vi "test_Add Command_Channel Reference Error.vi"(8 "error in (no error)":errorcluster, 11 "TestCase in":refnum<class "Instrument Addon Scripting API Messages Unit Tests.lvclass">) -> (0 "error out":errorcluster, 3 "TestCase out":refnum<class "Instrument Addon Scripting API Messages Unit Tests.lvclass">)   [LabVIEW 2019, in "Instrument Addon Scripting API Messages Unit Tests.lvclass"]
uses:
  Instrument Addon Scripting API Messages Unit Tests.lvclass
  APIs/Scripting API/TypeDefs/Command Settings.ctl
  <vilib>/NI VeriStand/Custom Device API/Custom Device Item Ref.ctl
  APIs/Scripting API/TypeDefs/Padding.ctl
  Instrument Addon Scripting API Messages Unit Tests.lvclass/Instrument Addon Scripting API Messages Unit Tests.ctl
  Addon/Addon Shared/SubVIs/Constants.vi
  <vilib>/NI/NI VeriStand Advanced SysDef API/_SubVIs/SysDef.Search.GUID.vi
  <vilib>/addons/_JKI Toolkits/VI Tester/TestCase.llb/TestCase.lvclass
  Instrument Addon Scripting API Test Assets/Instrument Addon Scripting API Test Assets.lvclass
  <vilib>/NI/NI VeriStand Advanced SysDef API/SysDef API/Advanced System Definition.lvlib
  Addon/Addon Shared/Instrument Addon Shared.lvlib
  <vilib>/NI VeriStand/Custom Device API/Custom Device API.lvlib
  APIs/Scripting API/Instrument Addon Scripting API.lvlib
  C:/Program Files (x86)/National Instruments/LabVIEW 2019/vi.lib/addons/_JKI Toolkits/VI Tester/TestCase.llb/TestCase.lvclass
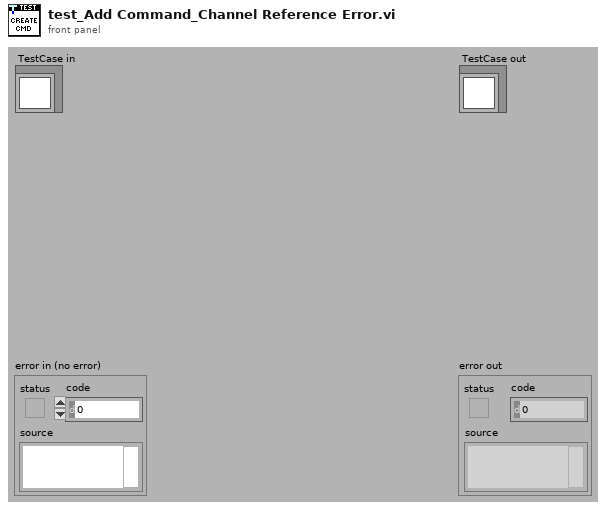
[diagram p1: front panel]
types:
  T1 = typedef "Custom Device API.lvlib/Custom Device Item Ref.ctl" = u64
  T2 = cluster{"Variable Name":string, "Channel Ref in":T1}
  T3 = typedef "Instrument Addon Scripting API.lvlib/Command Settings.ctl" = cluster{"Command Format":string, "Linked Channels":cluster{"Variable Name":string, "Channel Ref in":T1}[], "Use Padding?":bool, "Padding":T4}
  T4 = typedef "Instrument Addon Scripting API.lvlib/Padding.ctl" = cluster{"Pad Value":u8, "Length":u32}
  T5 = cluster{"Variable Name":string, "Channel Ref in":T1}[]
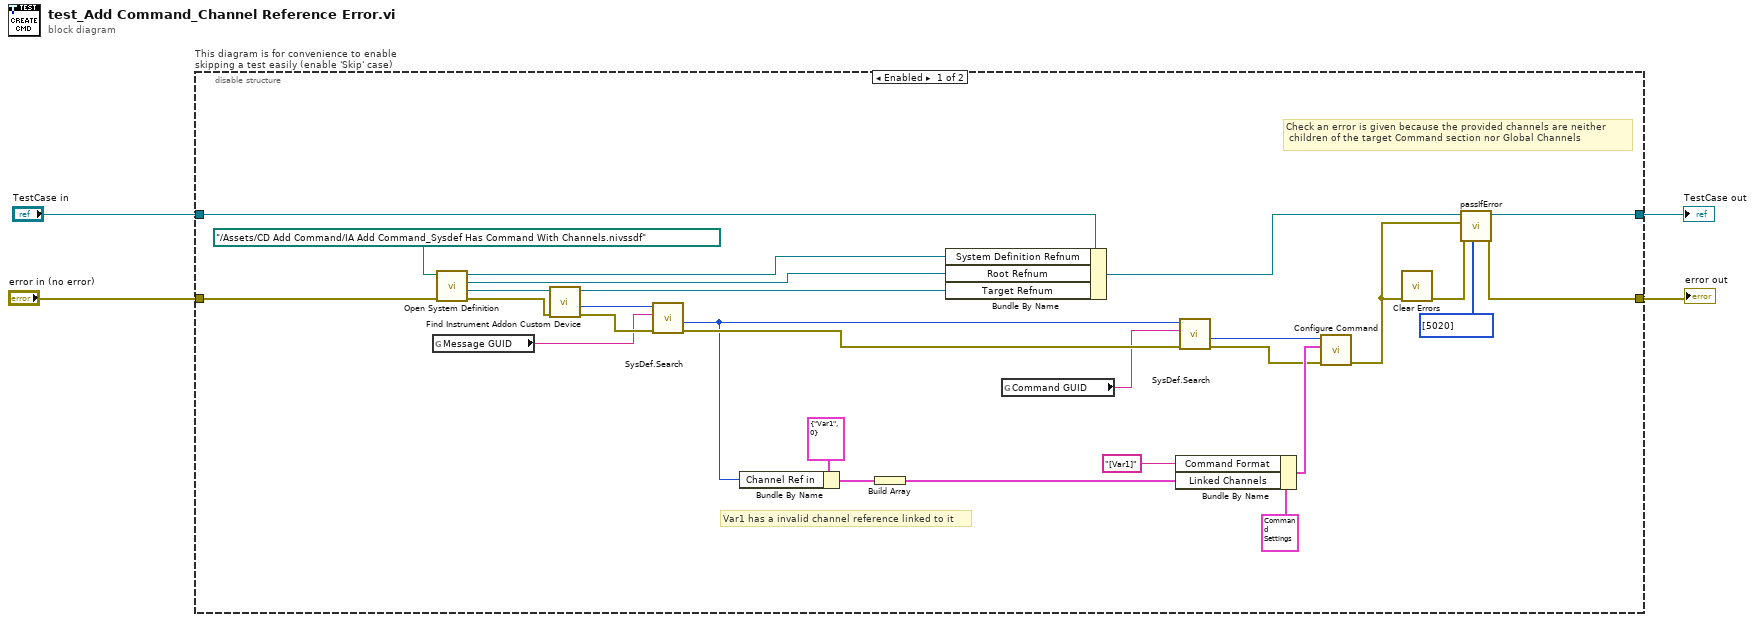
[diagram p0: block diagram]
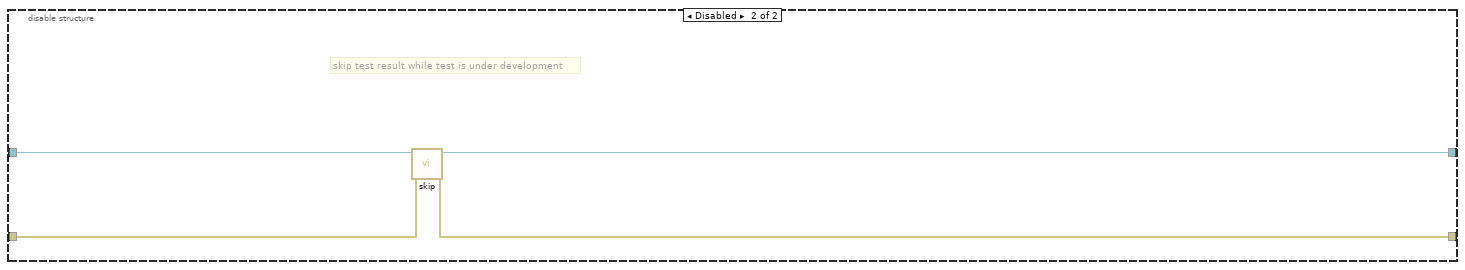
[diagram p2: hidden frame]
diagram:
  n1 = disable-structure "This diagram is for convenience to enable skipping a test easily (enable 'Skip' case)" shown="Enabled" {
    disable-tunnel: "TestCase in" -> [w19 w36]
    disable-tunnel: [w29 w34] -> w1
    disable-tunnel: [w30 w35] -> w3
    disable-tunnel: "error in (no error)" -> [w31 w33]
    frame Enabled {
      # "Var1 has a invalid channel reference linked to it"
      # "Check an error is given because the provided channels are neither\n children of the target Command section nor Global Channels"
      n2 = global read "Constants.vi" "Message GUID"() -> (w25:string)
      n3 = call "Open System Definition.vi"("error in (no error)"=w31, "System Definition File"=path "../Assets/CD Add Command/IA Add Command_Sysdef Has Command With Channels.nivssdf" ("SDF file")) -> ("error out"=w27:errorcluster, "Target Refnum"=w28:refnum<k24>, "Root Refnum"=w17:refnum<k24>, "System Definition Refnum"=w18:refnum<k24>)  [unwired: 6 in]
      n4 = call "Find Instrument Addon Custom Device.vi"("error in"=w27, "target in"=w28) -> ("error out"=w26:errorcluster, "NodeID"=w22:u64, "target out"=w16:refnum<k24>)  [unwired: 7 in]
      n5 = call-poly <vilib>:"SysDef.Search.vi"("error in (no error)"=w26, "GUID"=w25, "nodeID"=w22) -> ("error out"=w11:errorcluster, "Value out"=w7:u64)  [unwired: 5 in, 2 out]
      n6 = Bundle By Name(cluster=T2 {"Variable Name"="Var1", "Channel Ref in"=0} ("element"), "Channel Ref in"=w7) -> (w6:T2)
      n7 = Build Array(w6) -> (w5:T5)
      n8 = Bundle By Name(cluster=w19, "System Definition Refnum"=w18, "Root Refnum"=w17, "Target Refnum"=w16) -> (w15:refnum<class "Instrument Addon Scripting API Messages Unit Tests.lvclass">)
      n9 = global read "Constants.vi" "Command GUID"() -> (w9:string)
      n10 = Bundle By Name(cluster=T3 {"Command Format"="[Var1]+[Var2]", "Linked Channels"=[{"Variable Name"="Var1", "Channel Ref in"=32}, {"Variable Name"="Var2", "Channel Ref in"=33}], "Use Padding?"=FALSE, "Padding"={"Pad Value"=0, "Length"=0}} ("Settings"), "Command Format"="[Var1]", "Linked Channels"=w5) -> (w13:T3)
      n11 = call-poly <vilib>:"SysDef.Search.vi"("error in (no error)"=w11, "GUID"=w9, "nodeID"=w7) -> ("error out"=w10:errorcluster, "Value out"=w12:u64)  [unwired: 5 in, 2 out]
      n12 = call "Configure Command.vi"("error in (no error)"=w10, "settings"=w13, "command refnum in"=w12) -> ("error out"=w14:errorcluster)  [unwired: 7 in, 1 out]
      n13 = call <vilib>:"Clear Errors.vi"("error in (no error)"=w14) -> ("error out"=w20:errorcluster)  [unwired: 5 in, 1 out]
      n14 = call-dynamic "passIfError.vi"("passing error codes (default = any error code)"=i32[] [5020], "error in (no error)"=w20, "error"=w14, "TestCase in"=w15) -> ("error out"=w30:errorcluster, "TestCase out"=w29:refnum<class "Instrument Addon Scripting API Messages Unit Tests.lvclass">)  [unwired: 6 in]
    }
    frame Disabled {
      # "skip test result while test is under development"
      n15 = call <vilib>:"skip.vi"("error in (no error)"=w33, "TestCase in"=w36) -> ("error out"=w35:errorcluster, "TestCase out"=w34:refnum<class "Instrument Addon Scripting API Messages Unit Tests.lvclass">)  [unwired: 8 in]
    }
  }
  "error out" <- w3
  "TestCase out" <- w1
